vi "3.3v Output.vi"   [LabVIEW 2011]
uses:
  <vilib>/rvi/eio/common/nirviEmuTemplateMethod_errors.vi
  <vilib>/eio/EIONode/EIONode.xnode
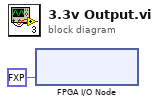
[diagram p0: block diagram]
diagram:
  n1 = xnode "FPGA I/O Node"("Mod3/AO0"=fxp<+/-,20,5> 3.0) -> ()  [unwired: 1 in, 1 out]
